vi "fit02.vi"(2 "input":T1) -> (0 "fitness":dbl=1.2)   [LabVIEW 2013]
uses:
  <vilib>/Analysis/Matrix/Datatypes/RealMatrix.ctl
  <vilib>/Analysis/Matrix/Numeric/Conversions/Matrix To Array - RM.vi
  <vilib>/Analysis/Matrix/NI_Matrix.lvlib
panel:
  out "subarray":dbl[](array[numeric])
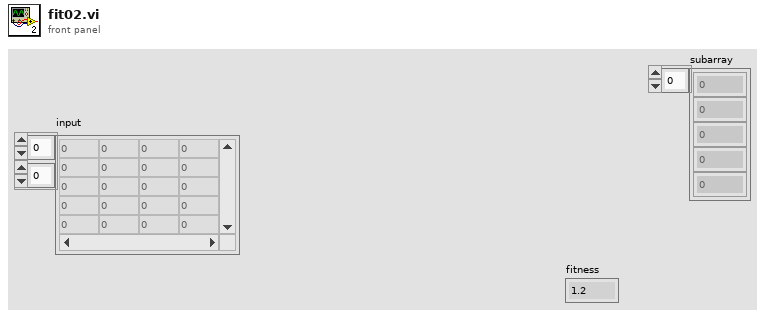
[diagram p1: front panel]
types:
  T1 = typedef "NI_Matrix.lvlib/RealMatrix.ctl" = dbl[][]
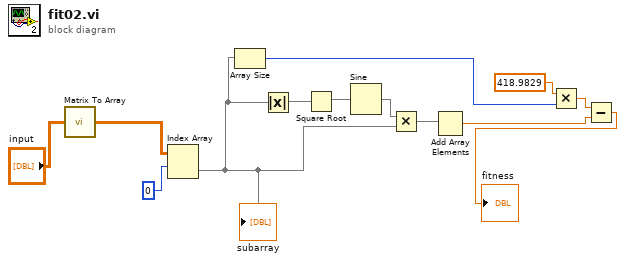
[diagram p0: block diagram]
diagram:
  n1 = call-poly <vilib>:"Matrix To Array.vi"("Real Matrix"="input") -> ("Real 2D Array"=w12:dbl[][])
  n2 = Index Array(array=w12, index (row)=0) -> (element=w5:dbl[])  [unwired: 1 in]
  "subarray" <- w5
  n3 = Array Size(array=w5) -> (size(s)=w4:i32)
  n4 = Absolute Value(x=w5) -> (abs(x)=w10:dbl[])
  n5 = Square Root(x=w10) -> (sqrt(x)=w9:dbl[])
  n6 = Sine(x=w9) -> (sin(x)=w8:dbl[])
  n7 = Multiply(x=w8, y=w5) -> (x*y=w7:dbl[])
  n8 = Add Array Elements(numeric array=w7) -> (sum=w2:dbl)
  n9 = Multiply(x=418.9829, y=w4) -> (x*y=w3:dbl)
  n10 = Subtract(x=w3, y=w2) -> (x-y=→"fitness":dbl)
